vi "Destroy Windows Message Queue.vi"(1 "error in (no error)":errorcluster, 2 "win msg queue":T1) -> (0 "error out":errorcluster)   [LabVIEW 2017, in "Windows messages for Labview (32 and 64).lvlib"]
doc: "Destroys and disposes of a windows message queue. This VI must be called before exiting a VI in which a windows message queue is used.\n\nParameters:\nwin msg queue: the queue to destroy.\n\nErrors:\nReturns 6751 if the queue is not a valid windows message queue."
uses:
  Windows messages for Labview (32 and 64).lvlib
  Win Msg Queue RefNum.ctl
  Windows Messages for LabVIEW_64.dll
  Windows Messages for LabVIEW_32.dll
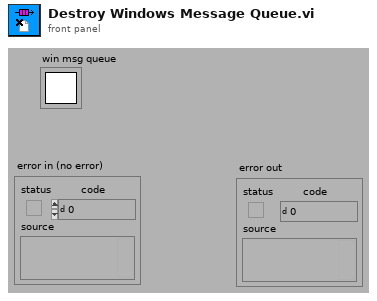
[diagram p1: front panel]
types:
  T1 = typedef "Windows messages for Labview (32 and 64).lvlib/Win Msg Queue RefNum.ctl" = refnum<k1>
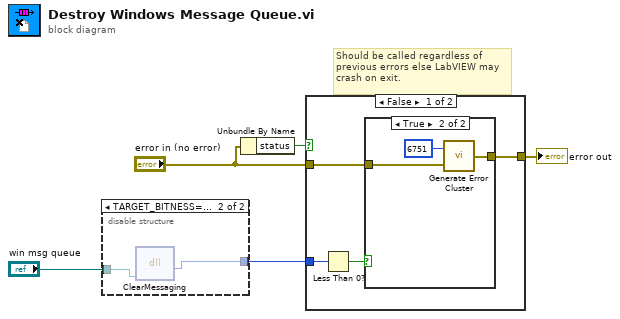
[diagram p0: block diagram]
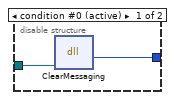
[diagram p2: hidden frame]
diagram:
  # "Should be called regardless of\nprevious errors else LabVIEW may\ncrash on exit."
  n1 = disable-structure shown="TARGET_BITNESS==32" {
    disable-tunnel: "win msg queue" -> [w7 w9]
    disable-tunnel: [w6 w8] -> w1
    frame condition #0 (active) {
      n2 = dll-call lib="M:/_dev/progs/LabVIEW/_lib/Windows Messages for Labview/llb/Windows Messages for LabVIEW_64.dll" fn="ClearMessaging"("occurrence"=w7) -> ("return type"=w6:i32)  [unwired: 4 in, 2 out]
    }
    frame condition #1 {
      n3 = dll-call lib="D:/labview_d/temp/Windows Messaging/Windows Messages for Labview/llb/Windows Messages for LabVIEW_32.dll" fn="ClearMessaging"("occurrence"=w9) -> ("return type"=w8:i32)  [unwired: 4 in, 2 out]
    }
  }
  n4 = Unbundle By Name("error in (no error)") -> ("status"=w3:bool)
  n5 = case shown="False" w3 {
    tunnel: "error in (no error)" -> [w13 w18]
    tunnel: [w11 w18] -> w4
    tunnel: w1 -> [w10 _]
    frame False {
      n6 = Less Than 0?(x=w10) -> (x < 0?=w12:bool)
      n7 = case shown="True" w12 {
        tunnel: w13 -> [w14 w16]
        tunnel: [w14 w17] -> w11
        frame False {
        }
        frame True {
          n8 = call "Generate Error Cluster.vi"("error in (no error)"=w16, "Error Code"=6751) -> ("error out"=w17:errorcluster)
        }
      }
    }
    frame True {
    }
  }
  "error out" <- w4
